vi "Get Hardware Parameter value from DB Array.vi"(9 "Parameter Name":string="Communication Type", 10 "Data Type":string(combo), 11 "Data":string[](array[string])) -> (1 "Enum& Ring":i32, 2 "Boolean":bool, 3 "String":string, 4 "Float & Nubmer":dbl, 5 "Unit":string)   [LabVIEW 2020]
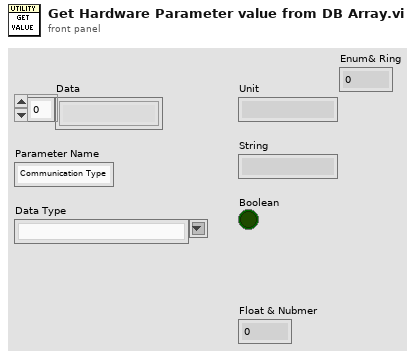
[diagram p1: front panel]
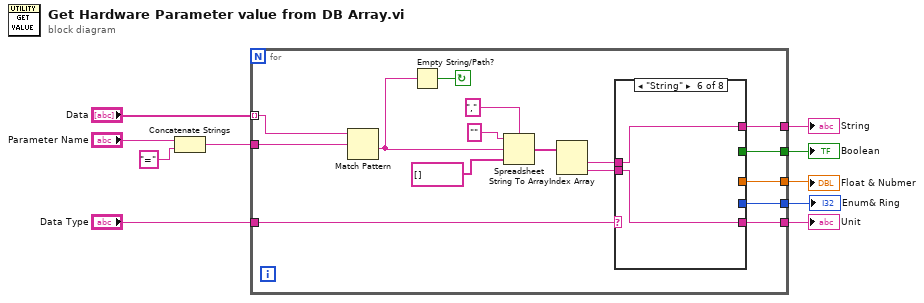
[diagram p0: block diagram]
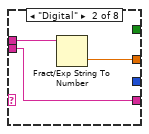
[diagram p3: hidden frame]
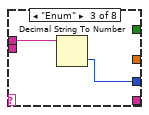
[diagram p4: hidden frame]
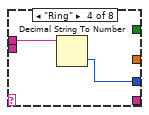
[diagram p5: hidden frame]
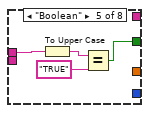
[diagram p6: hidden frame]
diagram:
  n1 = Concatenate Strings("Parameter Name", "=" ("string")) -> (w5:string)
  n2 = for {
    tunnel: "Data" -> [w26] mode=indexing
    tunnel: w5 -> [w25]
    tunnel: "Data Type" -> [w19]
    tunnel: [w16] -> w7
    tunnel: [w15] -> w8
    tunnel: [w14] -> w9
    tunnel: [w12] -> w10
    tunnel: [w11] -> w1
    stop <- w20 continue-if-true
    n3 = Match Pattern(string=w26, regular expression=w25) -> (after substring=w21:string)  [unwired: 1 in, 3 out]
    n4 = Empty String/Path?(string/path=w21) -> (empty?=w20:bool)
    n5 = Spreadsheet String To Array(delimiter (Tab)=",", format string="", spreadsheet string=w21, array type (2D Dbl)=string[] [] ("array w/ subset deleted")) -> (array=w22:string[])
    n6 = Index Array(array=w22) -> (element #1=w18:string, element #2=w13:string)  [unwired: 2 in]
    n7 = case shown="\"String\"" w19 {
      tunnel: w18 -> [_ w29 w31 w33 w37 w39 w40 _]
      tunnel: [_ _ _ _ w34 _ _ _] -> w16
      tunnel: [_ _ _ _ _ w39 w40 _] -> w15
      tunnel: [_ w28 _ _ _ _ _ _] -> w14
      tunnel: w13 -> [_ w27 _ _ _ w38 _ _]
      tunnel: [_ w27 _ _ _ w38 _ _] -> w12
      tunnel: [_ _ w30 w32 _ _ _ _] -> w11
      frame Default {
      }
      frame "Digital" {
        n8 = Fract/Exp String To Number(string=w29) -> (number=w28:dbl)  [unwired: 3 in, 1 out]
      }
      frame "Enum" {
        n9 = Decimal String To Number(string=w31) -> (number=w30:i32)  [unwired: 2 in, 1 out]
      }
      frame "Ring" {
        n10 = Decimal String To Number(string=w33) -> (number=w32:i32)  [unwired: 2 in, 1 out]
      }
      frame "Boolean" {
        n11 = To Upper Case(1:w37) -> (0:w36:string)
        n12 = Equal?(x=w36, y="TRUE") -> (x = y?=w34:bool)
      }
      frame "String" {
      }
      frame "VISAResourceName" {
      }
      frame "Array" {
      }
    }
  }
  "Boolean" <- w7
  "String" <- w8
  "Float & Nubmer" <- w9
  "Unit" <- w10
  "Enum& Ring" <- w1
